vi "Handle Command.vi"(8 "error in (no error)":errorcluster, 9 "Value":bool, 11 "Valve in":refnum<class "InterlockControl.lvclass">) -> (0 "error out":errorcluster, 3 "Valve out":refnum<class "InterlockControl.lvclass">)   [LabVIEW 2020, in "VolatusControl.lvlib" / "InterlockControl.lvclass"]
uses:
  InterlockControl.lvclass
  InterlockControl.lvclass/InterlockControl.ctl
  Interlock Action.ctl
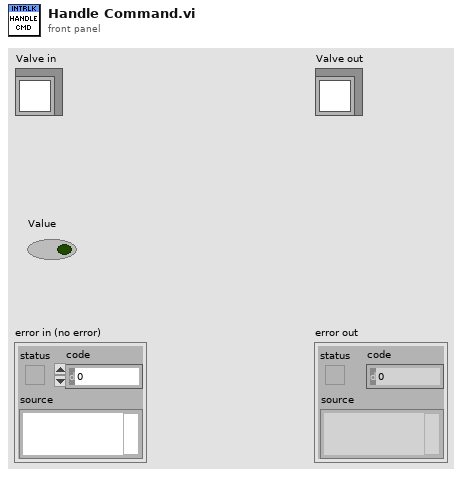
[diagram p1: front panel]
types:
  T1 = typedef "VolatusControl.lvlib/InterlockControl.lvclass/Interlock Action.ctl" = enum16{"None", "Cmd False", "Cmd True"}
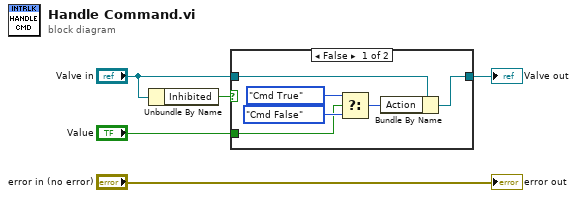
[diagram p0: block diagram]
diagram:
  n1 = Unbundle By Name("Valve in") -> ("Inhibited"=w4:bool)
  n2 = case shown="False" w4 {
    tunnel: "Valve in" -> [w11 w12]
    tunnel: "Value" -> [w8 _]
    tunnel: [w6 w12] -> w1
    frame False {
      n3 = Select(t=Interlock_Action."Cmd True" ("Action"), s=w8, f=Interlock_Action."Cmd False" ("Action")) -> (s? t:f=w7:T1)
      n4 = Bundle By Name(cluster=w11, "Action"=w7) -> (w6:refnum<class "InterlockControl.lvclass">)
    }
    frame True {
    }
  }
  "Valve out" <- w1
  "error out" <- "error in (no error)"
